vi "DAQ_DC Voltage Gen Close.vi"(0 "DAQmx Task In":refnum<k21>, 11 "error in":errorcluster) -> (15 "error out":errorcluster)   [LabVIEW 2021, in "DAQ_DC Voltage Generation.lvlib"]
doc: "Aborts and clears the DC Voltage Generation Task"
uses:
  DAQ_DC Voltage Generation.lvlib
panel:
  # "Inputs"
  # "Outputs"
  # "Overview:\nThis VI closes the DC Voltage Generation task\n\nHardware Requirement: A compatible PXI, PCIe, USB, cDAQ or Testscale device\n\nSoftware Requirement: NI DAQmx 2022 Q4 or later\n\nInstructions:\n1. Input the DC Voltage Generation task through DAQmx Task In control\n2. This VI aborts and clears the DAQmx Task"
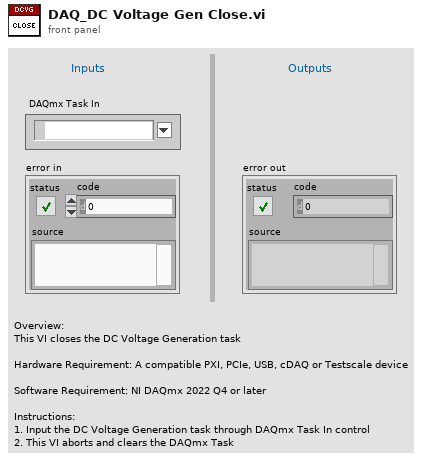
[diagram p1: front panel]
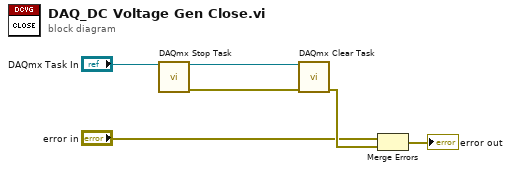
[diagram p0: block diagram]
diagram:
  n1 = call <vilib>:"DAQmx Stop Task.vi"("task/channels in"="DAQmx Task In") -> ("task out"=w6:refnum<k21>, "error out"=w5:errorcluster)  [unwired: 13 in]
  n2 = call <vilib>:"DAQmx Clear Task.vi"("task in"=w6, "error in"=w5) -> ("error out"=w3:errorcluster)  [unwired: 13 in]
  n3 = Merge Errors("error in", w3) -> (→"error out":errorcluster)
